vi "PopulateChannelSettingsArray.vi"(1 "Update size?":bool=TRUE, 2 "error in":errorcluster, 3 "Input arm settings ref":refnum<vi>, 4 "Enum in":refnum<vi>) -> (0 "error out":errorcluster)   [LabVIEW 2015]
doc: "Populates the channel selection array with options for channels"
uses:
  controls/ChannelSettings.ctl
panel:
  in  "Input arm default settings":T1={"Convert?"=FALSE, "Config"={"Vref"=1.25, "Rgain"=100000.0, "Rset"=10000.0, "Rseries"=1000.0, "Input polarity?"=FALSE}}
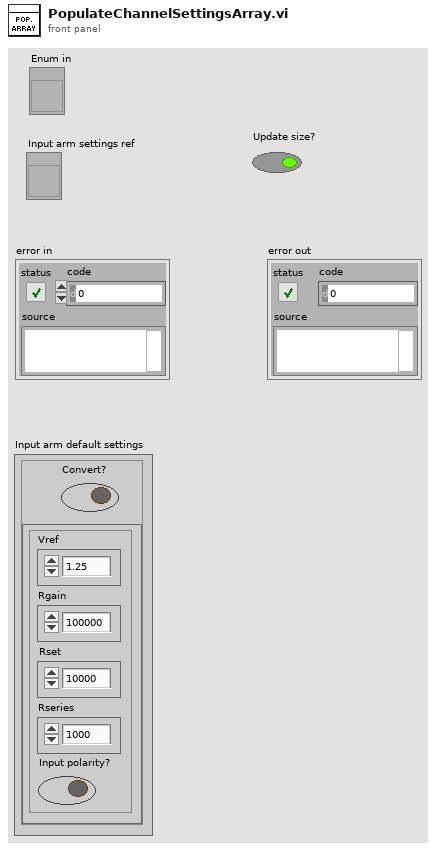
[diagram p1: front panel]
types:
  T1 = typedef "ChannelSettings.ctl" = cluster{"Convert?":bool, "Config":cluster{"Vref":dbl, "Rgain":dbl, "Rset":dbl, "Rseries":dbl, "Input polarity?":bool}}
  T2 = cluster{string, u16, "Input arm default settings":T1}
  T3 = cluster{"Enum string":string, "Enum ID":i16, "Input arm settings":T1}[]
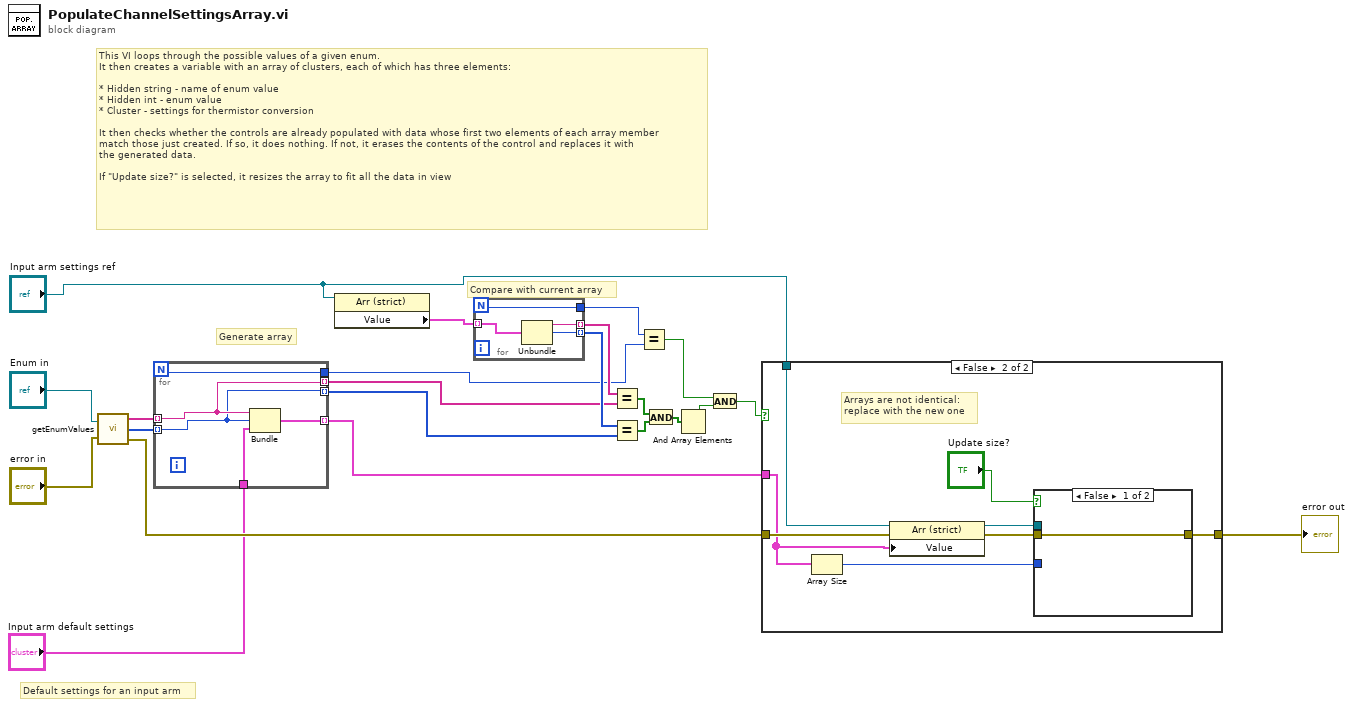
[diagram p0: block diagram]
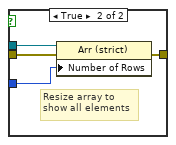
[diagram p3: hidden frame]
diagram:
  # "Default settings for an input arm"
  # "Compare with current array"
  # "Generate array"
  # "This VI loops through the possible values of a given enum.\nIt then creates a variable with an array of clusters, each of which has three elements:\n\n* Hidden string - name of enum value\n* Hidden int - enum value\n* Cluster - settings for thermistor conversion\n\nIt then checks whether the controls are already populated with data whose first two elements of each array member\nmatch those just created. If so, it does nothing. If not, it erases the contents of the control and replaces it with \nthe generated data.\n\nIf \"Update size?\" is selected, it resizes the array to fit all the data in view"
  n1 = call "getEnumValues.vi"("Enum reference"="Enum in", "error in (no error)"="error in") -> ("Enum labels"=w19:string[], "Enum values"=w18:u16[], "error out"=w22:errorcluster)
  n2 = for {
    N -> [w24]
    tunnel: w19 -> [w26] mode=indexing
    tunnel: w18 -> [w25] mode=indexing
    tunnel: [w27] -> w11 mode=indexing
    tunnel: [w26] -> w4 mode=indexing
    tunnel: [w25] -> w3 mode=indexing
    tunnel: [w24] -> w9
    tunnel: "Input arm default settings" -> [w23]
    n3 = Bundle(w26, w25, "Input arm default settings"=w23) -> (w27:T2)  [unwired: 1 in]
  }
  n4 = property class="Arr (strict)"(reference="Input arm settings ref") -> ("Value"=w17:T3)  [unwired: 1 in, 2 out]
  n5 = for {
    N -> [w28]
    tunnel: w17 -> [w31] mode=indexing
    tunnel: [w30] -> w16 mode=indexing
    tunnel: [w29] -> w15 mode=indexing
    tunnel: [w28] -> w10
    n6 = Unbundle(w31) -> ("Enum string"=w30:string, "Enum ID"=w29:i16)  [unwired: 1 out]
  }
  n7 = Equal?(x=w16, y=w4) -> (x = y?=w14:bool[])
  n8 = Equal?(x=w15, y=w3) -> (x = y?=w2:bool[])
  n9 = Equal?(x=w10, y=w9) -> (x = y?=w7:bool)
  n10 = And(x=w14, y=w2) -> (x .and. y?=w13:bool[])
  n11 = And Array Elements(Boolean array=w13) -> (logical AND=w8:bool)
  n12 = And(x=w7, y=w8) -> (x .and. y?=w6:bool)
  n13 = case shown="False" w6 {
    tunnel: w22 -> [w32 w40]
    tunnel: "Input arm settings ref" -> [_ w39]
    tunnel: [w32 w35] -> w12
    tunnel: w11 -> [_ w33]
    frame True {
      # "Arrays are identical: don't update anything"
      # "Resize array to show all elements"
    }
    frame False {
      # "Arrays are not identical:\nreplace with the new one"
      n14 = Array Size(array=w33) -> (size(s)=w36:i32)
      n15 = property on="Property Node" class="Arr (strict)"(reference=w39, error in=w40, "Value"=w33) -> (reference out=w37:refnum<vi>, error out=w38:errorcluster)
      n16 = case shown="False" "Update size?" {
        tunnel: w38 -> [w41 w45]
        tunnel: w37 -> [_ w44]
        tunnel: w36 -> [_ w42]
        tunnel: [w41 w43] -> w35
        frame False {
        }
        frame True {
          # "Resize array to\nshow all elements"
          n17 = property on="Property Node" class="Arr (strict)"(reference=w44, error in=w45, "Number of Rows"=w42) -> (error out=w43:errorcluster)  [unwired: 1 out]
        }
      }
    }
  }
  "error out" <- w12
